vi "Test XY Graph with TipStrip.vi"() -> ()   [LabVIEW 2019, in "XY Graph Add-Ons.lvlib"]
uses:
  XY Graph Add-Ons.lvlib
  XY Graph Refnum.ctl
panel:
  out "XY Graph TipStrip":string
  out "XY Graph":cluster{dbl[], dbl[]}[](graph)
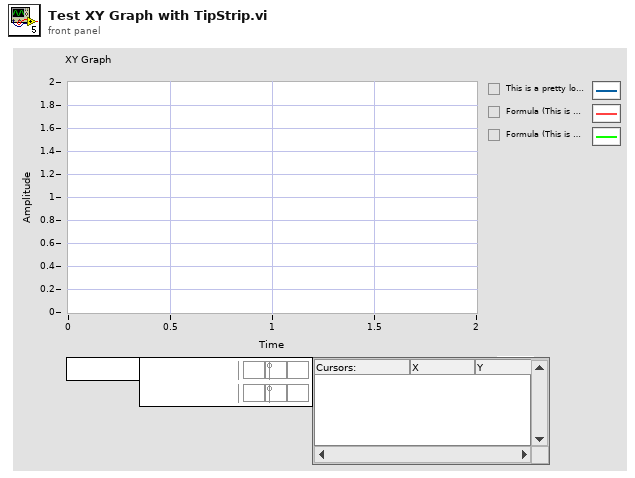
[diagram p1: front panel]
types:
  T1 = cluster{"XY Graph TipStrip":refnum<event-registration>}
  T2 = typedef "XY Graph Add-Ons.lvlib/XY Graph Tool Panels Visibility.ctl" = cluster{"Scale Legend Vis":bool, "X-Scrollbar Vis":bool, "Cursor Panel Vis":bool, "Graph Palette Vis":bool}
  T3 = typedef "LVPoint32TypeDef.ctl" = cluster{"Horizontal":i32, "Vertical":i32}
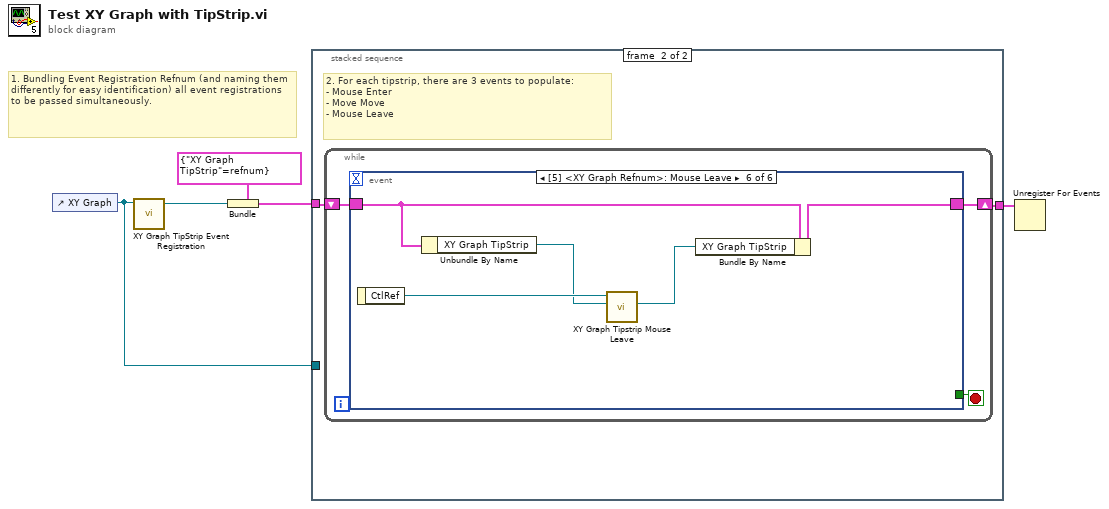
[diagram p0: block diagram]
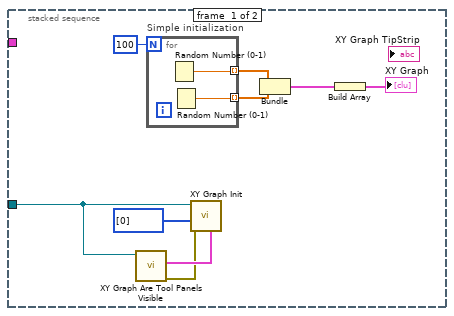
[diagram p2: hidden frame]
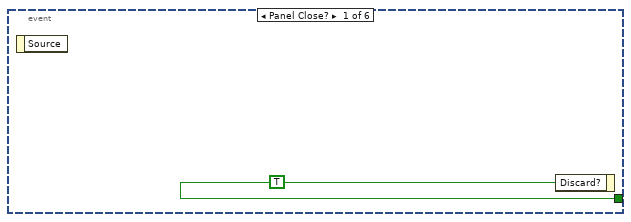
[diagram p3: hidden frame]
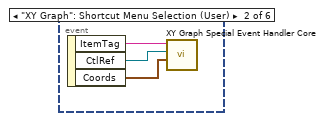
[diagram p4: hidden frame]
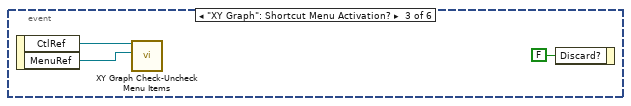
[diagram p5: hidden frame]
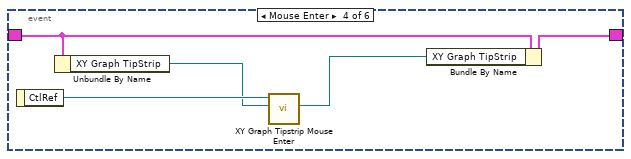
[diagram p6: hidden frame]
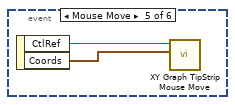
[diagram p7: hidden frame]
diagram:
  # "1. Bundling Event Registration Refnum (and naming them differently for easy identification) all event registrations to be passed simultaneously."
  n1 = control-ref of="XY Graph"() -> (w2:refnum<vi>)
  n2 = call "XY Graph TipStrip Event Registration.vi"("XY Graph Refnum"=w2) -> ("Event Registration Refnum"=w5:refnum<event-registration>)  [unwired: 8 in, 2 out]
  n3 = Bundle(cluster=T1 {"XY Graph TipStrip"=refnum} ("Event Registration Refnums"), "XY Graph TipStrip"=w5) -> (w3:T1)
  n4 = stacked-sequence {
    tunnel: [_ w18] -> w4
    tunnel: w3 -> [_ w17]
    tunnel: w2 -> [w8 _]
    frame #0 {
      n5 = call "XY Graph Are Tool Panels Visible.vi"("XY Graph Ref"=w8) -> ("Error Out"=w6:errorcluster, "Graph Tool Panels Visibility"=w7:T2)  [unwired: 8 in, 1 out]
      n6 = for "Simple initialization" {
        N: 100 -> [_]
        tunnel: [w16] -> w12 mode=indexing
        tunnel: [w15] -> w13 mode=indexing
        n7 = Random Number (0-1)() -> (number: 0 to 1=w16:dbl)
        n8 = Random Number (0-1)() -> (number: 0 to 1=w15:dbl)
      }
      n9 = call "XY Graph Init.vi"("Graph Tool Panels Visibility"=w7, "Error In"=w6, "Plots to Skip (none)"=i32[] [0], "XYGraph in"=w8) -> ()  [unwired: 7 in, 1 out]
      n10 = Bundle(w12, w13) -> (w14:cluster{dbl[], dbl[]})  [unwired: 1 in]
      n11 = Build Array(w14) -> (→"XY Graph":cluster{dbl[], dbl[]}[])
    }
    frame #1 {
      # "2. For each tipstrip, there are 3 events to populate:\n- Mouse Enter\n- Move Move\n- Mouse Leave"
      n12 = while {
        shift-right: [w19] -> w18
        shift-left: w17 -> [w21]
        stop <- w20 stop-if-true
        n13 = event shown="[5] <XY Graph Refnum>: Mouse Leave" {
          selector: w21 -> [_ _ _ w31 _ w37]
          dyn-events: [_ _ _ w33 _ w36] -> w19
          timeout: _ -> [_ _ _ _ _ _]
          tunnel: [w22 _ _ _ _ _] -> w20
          event Panel Close? {
            w22 = TRUE ("Discard?")
            n14 = event-data() -> ()  [unwired: 1 in, 1 out]
            n15 = event-data("Discard?"=w22) -> ()  [unwired: 1 in, 1 out]
          }
          event "XY Graph": Shortcut Menu Selection (User) {
            n16 = event-data() -> ("ItemTag"=w25:string, "CtlRef"=w24:refnum<vi>, "Coords"=w23:T3)  [unwired: 1 in]
            n17 = call "XY Graph Special Event Handler Core.vi"("Coords"=w23, "XYGraph in"=w24, "ItemTag"=w25) -> ()  [unwired: 7 in, 2 out]
          }
          event "XY Graph": Shortcut Menu Activation? {
            n18 = event-data() -> ("CtlRef"=w27:refnum<vi>, "MenuRef"=w26:refnum<k9>)  [unwired: 1 in]
            n19 = call "XY Graph Check-Uncheck Menu Items.vi"("Menu in"=w26, "XY Graph Refnum"=w27) -> ()  [unwired: 8 in, 2 out]
            n20 = event-data("Discard?"=FALSE) -> ()  [unwired: 1 in, 1 out]
          }
          event Mouse Enter {
            n21 = event-data() -> ("CtlRef"=w32:refnum<vi>)  [unwired: 1 in]
            n22 = Unbundle By Name(w31) -> ("XY Graph TipStrip"=w30:refnum<event-registration>)
            n23 = call "XY Graph Tipstrip Mouse Enter.vi"("Event Registration Refnum"=w30, "XY Graph Refnum"=w32) -> ("Event Registration Refnum"=w29:refnum<event-registration>)  [unwired: 8 in, 1 out]
            n24 = Bundle By Name(cluster=w31, "XY Graph TipStrip"=w29) -> (w33:T1)
          }
          event Mouse Move {
            n25 = event-data() -> ("CtlRef"=w35:refnum<vi>, "Coords"=w34:T3)  [unwired: 1 in]
            n26 = call "XY Graph TipStrip Mouse Move.vi"("Coords"=w34, "XY Graph Refnum"=w35) -> ()  [unwired: 7 in, 3 out]
          }
          event Mouse Leave {
            n27 = event-data() -> ("CtlRef"=w40:refnum<vi>)  [unwired: 1 in]
            n28 = Unbundle By Name(w37) -> ("XY Graph TipStrip"=w39:refnum<event-registration>)
            n29 = call "XY Graph Tipstrip Mouse Leave.vi"("Event Registration Refnum"=w39, "XY Graph Refnum"=w40) -> ("Event Registration Refnum"=w38:refnum<event-registration>)  [unwired: 8 in, 1 out]
            n30 = Bundle By Name(cluster=w37, "XY Graph TipStrip"=w38) -> (w36:T1)
          }
        }
      }
    }
  }
  n31 = Unregister For Events(event registration refnum=w4) -> ()  [unwired: 1 in, 1 out]
